vi "Swerve Calibrate.vi"(8 "error in (no error)":errorcluster, 11 "Wheel Corner":T1(ring)) -> (0 "error out":errorcluster)   [LabVIEW 2016]
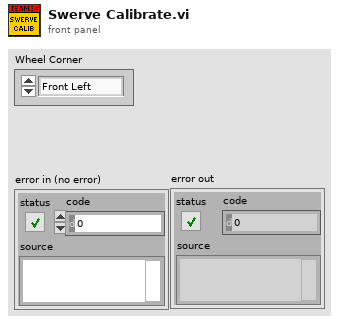
[diagram p1: front panel]
types:
  T1 = enum16{"Front Left", "Front Right", "Back Left", "Back Right"}
  T2 = typedef "WPI_SwitchDevRef.ctl" = cluster{"DevStatus":errorcluster, "DIO Channel":T3, "CntIndex":T4, "Normally Closed":bool}
  T3 = typedef "FPGA_DIOChannel.ctl" = enum8{"DIO 0", "DIO 1", "DIO 2", "DIO 3", "DIO 4", "DIO 5", "DIO 6", "DIO 7", "DIO 8", "DIO 9", "DIO MXP 0", "DIO MXP 1", "DIO MXP 2", "DIO MXP 3", "DIO MXP 4", "DIO MXP 5", "DIO MXP 6", "DIO MXP 7", "DIO MXP 8", "DIO MXP 9", "DIO MXP 10", "DIO MXP 11", "DIO MXP 12", "DIO MXP 13", "DIO MXP 14", "DIO MXP 15", "SPI Port CS1", "SPI Port CS2", "SPI Port CS3", "SPI Port MISO", "SPI Port MOSI", "Invalid"}
  T4 = typedef "FPGA_CounterCtrSystemIndex.ctl" = enum8{"Ctr 0", "Ctr 1", "Ctr 2", "Ctr 3", "Ctr 4", "Ctr 5", "Ctr 6", "Ctr 7", "Invalid"}
  T5 = typedef "WPI_MotorControlDeviceRef.ctl" = cluster{"DeviceStatus":errorcluster, "Type":T6, "PWM":cluster{"PWM Channel":T7, "DeadBand":T8}, "CAN":cluster{"Device Number":u8, "SetOutput VI Ref":variant, "GetOutput VI Ref":variant, "Enable VI Ref":variant, "Disable VI Ref":variant, "Data":variant}, "Invert":bool}
  T6 = typedef "WPI_MotorControlType.ctl" = enum16{"PWM", "CAN"}
  T7 = typedef "FPGA_DIOPWMChannel.ctl" = enum8{"PWM 0", "PWM 1", "PWM 2", "PWM 3", "PWM 4", "PWM 5", "PWM 6", "PWM 7", "PWM 8", "PWM 9", "PWM MXP 0", "PWM MXP 1", "PWM MXP 2", "PWM MXP 3", "PWM MXP 4", "PWM MXP 5", "PWM MXP 6", "PWM MXP 7", "PWM MXP 8", "PWM MXP 9", "Invalid"}
  T8 = typedef "WPI_PWMDeadband.ctl" = cluster{"Name":string, "maxPositivePwm":i32, "minPositivePwm":i32, "centerPwm":i32, "maxNegativePwm":i32, "minNegativePwm":i32, "angularRange":u16}
  T9 = typedef "WPI_EncoderDevRef.ctl" = cluster{"DevStatus":errorcluster, "EncoderIndex":T10, "CounterIndex":T4, "DistancePerCount":dbl, "Decoding Type":T11}
  T10 = typedef "FPGA_EncoderIdx.ctl" = enum8{"Enc 0", "Enc 1", "Enc 2", "Enc 3", "Enc 4", "Enc 5", "Enc 6", "Enc 7", "Invalid"}
  T11 = typedef "WPI_EncoderType.ctl" = enum16{"1x", "2x", "4x"}
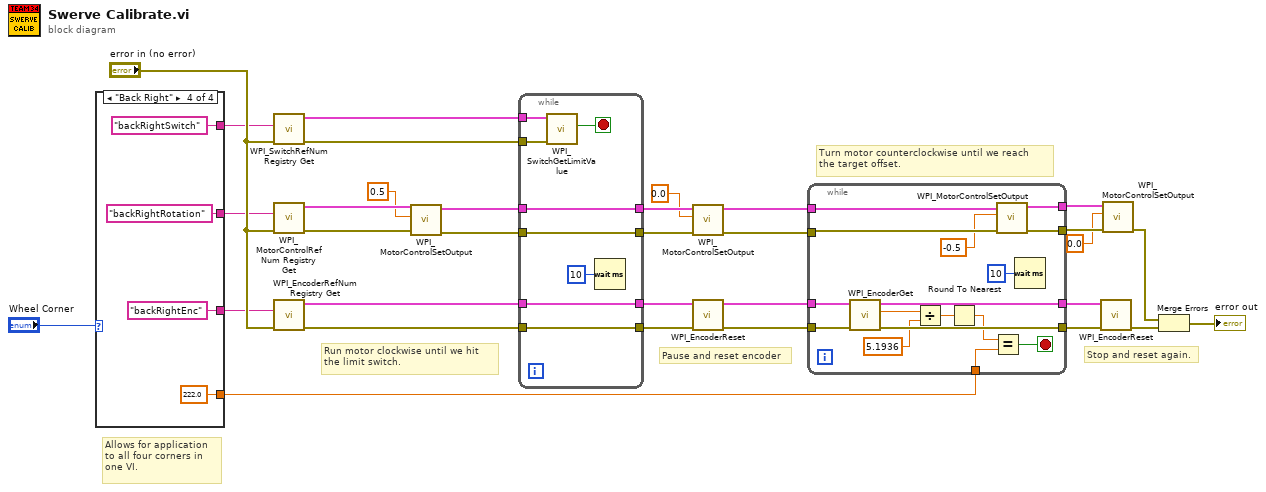
[diagram p0: block diagram]
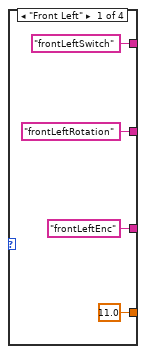
[diagram p2: hidden frame]
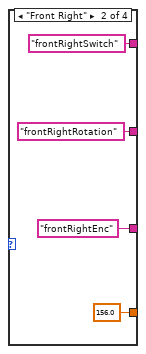
[diagram p3: hidden frame]
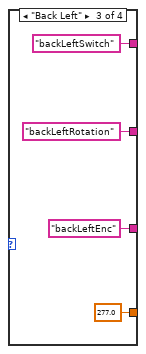
[diagram p4: hidden frame]
diagram:
  # "Allows for application\nto all four corners in \none VI."
  # "Stop and reset again."
  # "Turn motor counterclockwise until we reach\nthe target offset."
  # "Pause and reset encoder"
  # "Run motor clockwise until we hit\nthe limit switch."
  n1 = case shown="\"Back Right\"" "Wheel Corner" {
    tunnel: ["frontLeftSwitch" ("refnum name") "frontRightSwitch" ("refnum name") "backLeftSwitch" ("refnum name") "backRightSwitch" ("refnum name")] -> w5
    tunnel: ["frontLeftRotation" ("refnum name") "frontRightRotation" ("refnum name") "backLeftRotation" ("refnum name") "backRightRotation" ("refnum name")] -> w4
    tunnel: ["frontLeftEnc" ("refnum name") "frontRightEnc" ("refnum name") "backLeftEnc" ("refnum name") "backRightEnc" ("refnum name")] -> w3
    tunnel: [11.0 156.0 277.0 222.0] -> w1
    frame "Front Left" {
    }
    frame "Front Right" {
    }
    frame "Back Left" {
    }
    frame "Back Right" {
    }
  }
  n2 = call <vilib>:"WPI_SwitchRefNum Registry Get.vi"("error in (no error)"="error in (no error)", "refnum name"=w5) -> ("error out"=w27:errorcluster, "SwitchDevRef"=w28:T2)  [unwired: 8 in]
  n3 = call <vilib>:"WPI_MotorControlRefNum Registry Get.vi"("error in (no error)"="error in (no error)", "refnum name"=w4) -> ("error out"=w32:errorcluster, "MotorControlDevRef"=w31:T5)  [unwired: 8 in]
  n4 = call <vilib>:"WPI_EncoderRefNum Registry Get.vi"("error in (no error)"="error in (no error)", "refnum name"=w3) -> ("error out"=w20:errorcluster, "EncoderDevRef"=w21:T9)  [unwired: 8 in]
  n5 = call <vilib>:"WPI_MotorControlSetOutput.vi"("error in (no error)"=w32, "Output"=0.5 ("MotorOutput"), "MotorControlDevRef"=w31) -> ("error out"=w30:errorcluster, "MotorControlDevRef"=w29:T5)  [unwired: 6 in, 1 out]
  n6 = while {
    tunnel: w30 -> [w53]
    tunnel: w29 -> [w52]
    tunnel: w28 -> [w55]
    tunnel: w27 -> [w56]
    tunnel: [w53] -> w24
    tunnel: [w52] -> w26
    tunnel: [w51] -> w19
    tunnel: w21 -> [w51]
    tunnel: [w50] -> w18
    tunnel: w20 -> [w50]
    stop <- w54 stop-if-true
    n7 = call <vilib>:"WPI_SwitchGetLimitValue.vi"("error in (no error)"=w56, "SwitchDevRef"=w55) -> ("Switch Pressed"=w54:bool)  [unwired: 7 in, 2 out]
    n8 = Wait (ms)(milliseconds to wait=u32 10) -> ()  [unwired: 1 out]
  }
  n9 = call <vilib>:"WPI_MotorControlSetOutput.vi"("error in (no error)"=w24, "Output"=0.0, "MotorControlDevRef"=w26) -> ("error out"=w22:errorcluster, "MotorControlDevRef"=w23:T5)  [unwired: 6 in, 1 out]
  n10 = call <vilib>:"WPI_EncoderReset.vi"("error in (no error)"=w18, "EncoderDevRef"=w19) -> ("error out"=w16:errorcluster, "EncoderDevRef"=w17:T9)  [unwired: 8 in]
  n11 = while {
    tunnel: w17 -> [w72]
    tunnel: w16 -> [w71]
    tunnel: w23 -> [w70]
    tunnel: w22 -> [w69]
    tunnel: [w66] -> w14
    tunnel: [w65] -> w15
    tunnel: [w64] -> w13
    tunnel: [w63] -> w12
    tunnel: w1 -> [w60]
    stop <- w67 stop-if-true
    n12 = call <vilib>:"WPI_EncoderGet.vi"("error in (no error)"=w71, "EncoderDevRef"=w72) -> ("error out"=w66:errorcluster, "Distance"=w58:dbl, "EncoderDevRef"=w65:T9)  [unwired: 4 in, 3 out]
    n13 = Divide(x=w58, y=5.1936) -> (x/y=w57:dbl)
    n14 = Round To Nearest(number=w57) -> (nearest integer value=w62:dbl)
    n15 = Equal?(x=w62, y=w60) -> (x = y?=w67:bool)
    n16 = call <vilib>:"WPI_MotorControlSetOutput.vi"("error in (no error)"=w69, "Output"=-0.5, "MotorControlDevRef"=w70) -> ("error out"=w63:errorcluster, "MotorControlDevRef"=w64:T5)  [unwired: 6 in, 1 out]
    n17 = Wait (ms)(milliseconds to wait=u32 10) -> ()  [unwired: 1 out]
  }
  n18 = call <vilib>:"WPI_EncoderReset.vi"("error in (no error)"=w14, "EncoderDevRef"=w15) -> ("error out"=w8:errorcluster)  [unwired: 8 in, 1 out]
  n19 = call <vilib>:"WPI_MotorControlSetOutput.vi"("error in (no error)"=w12, "Output"=0.0, "MotorControlDevRef"=w13) -> ("error out"=w9:errorcluster)  [unwired: 6 in, 2 out]
  n20 = Merge Errors(w9, w8) -> (→"error out":errorcluster)
